vi "Configure Marker Out.vi"(1 "Marker Mode":u8(ring) items=["Fixed Low", "Fixed High", "Automatic", "Replicate Digital 0"], 2 "Selection Voltage":u8(ring) items=["Value", "Minimum", "Maximum", "Default"], 4 "Selection Skew":u8(ring) items=["Value", "Minimum", "Maximum", "Default"], 5 "Skew (s)":dbl, 6 "error in (no error)":errorcluster, 7 "Voltage Level (V)":dbl=1.0, 8 "Marker (0: Marker 1)":u16(ring) items=["Marker 1", "Marker 2", "Marker 3", "Marker 4"], 9 "VISA resource name":refnum<visa-resource-name>) -> (0 "error out":errorcluster, 3 "VISA resource name out":refnum<visa-resource-name>)   [LabVIEW 2020, in "Active Technologies AWG3000.lvlib"]
uses:
  Active Technologies AWG3000.lvlib
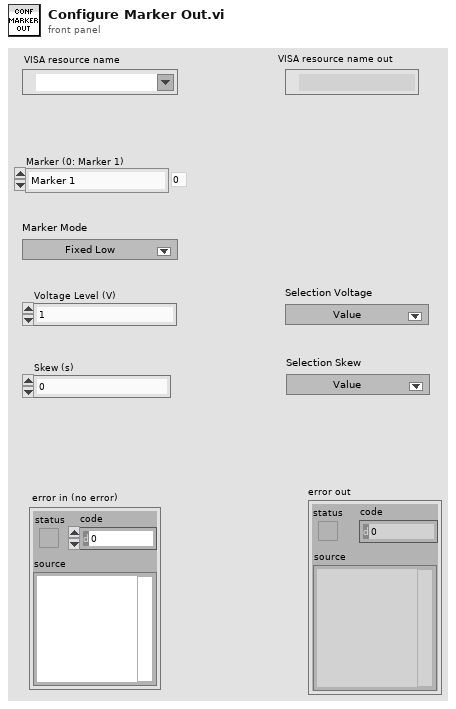
[diagram p1: front panel]
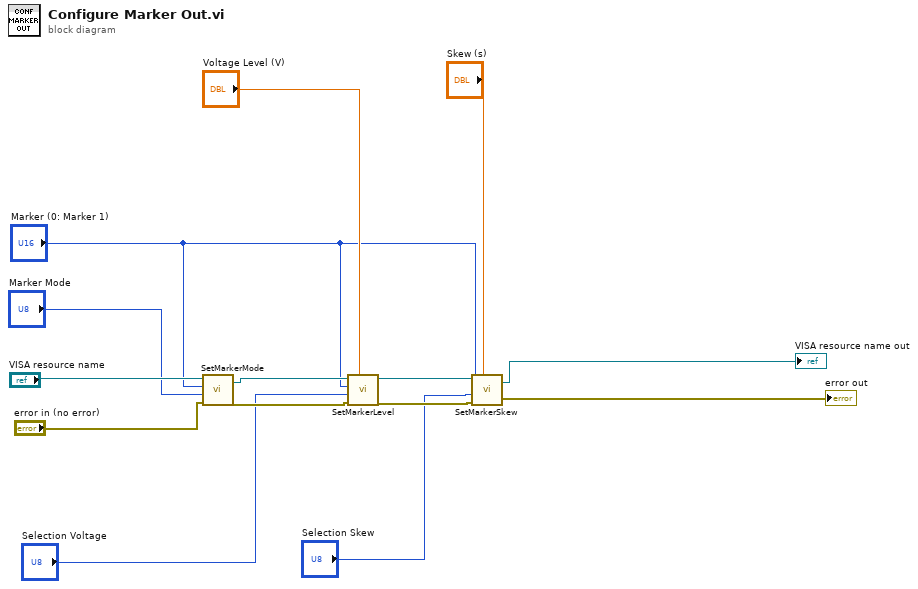
[diagram p0: block diagram]
diagram:
  n1 = call "SetMarkerMode.vi"("error in (no error)"="error in (no error)", "Marker Mode"="Marker Mode", "Marker (0: Marker 1)"="Marker (0: Marker 1)", "VISA resource name"="VISA resource name") -> ("error out"=w13:errorcluster, "VISA resource name out"=w14:refnum<visa-resource-name>)
  n2 = call "SetMarkerLevel.vi"("VISA resource name"=w14, "Marker (0: Marker 1)"="Marker (0: Marker 1)", "Selection"="Selection Voltage", "error in (no error)"=w13, "Voltage Level (V)"="Voltage Level (V)") -> ("VISA resource name out"=w11:refnum<visa-resource-name>, "error out"=w12:errorcluster)
  n3 = call "SetMarkerSkew.vi"("VISA resource name"=w11, "Marker (0: Marker 1)"="Marker (0: Marker 1)", "Selection"="Selection Skew", "error in (no error)"=w12, "Skew (s)"="Skew (s)") -> ("VISA resource name out"=→"VISA resource name out":refnum<visa-resource-name>, "error out"=→"error out":errorcluster)
